vi "Pack for gRPC.vi"(8 "error in":errorcluster, 9 "configuration / results":enum16{"Configuration", "Results"}(ring), 10 "data value":variant, 11 "measurement plugin service in":refnum<class "Measurement Plugin Service.lvclass">) -> (0 "error out":errorcluster, 2 "any":T1, 3 "measurement plugin service out":refnum<class "Measurement Plugin Service.lvclass">)   [LabVIEW 2021, in "NI Measurement Plug-In SDK.lvlib" / "Measurement Plugin Service.lvclass"]
uses:
  Measurement Plugin Service.lvclass
  <vilib>/gRPC/LabVIEW gRPC Library/Shared/Any.ctl
  <vilib>/gRPC/LabVIEW gRPC Library/grpc-lvsupport-release.lvlib
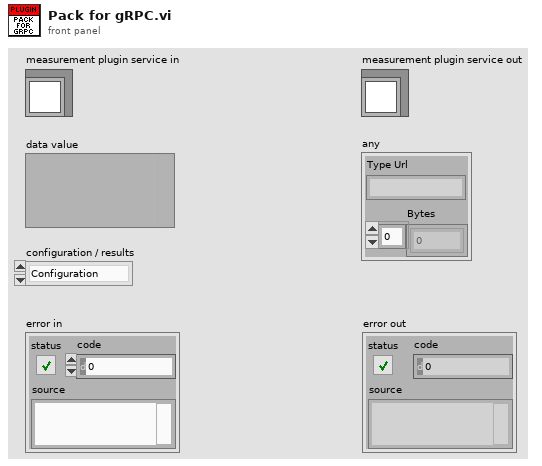
[diagram p1: front panel]
types:
  T1 = typedef "grpc-lvsupport-release.lvlib/Any.ctl" = cluster{"Type Url":string, "Bytes":u8[]}
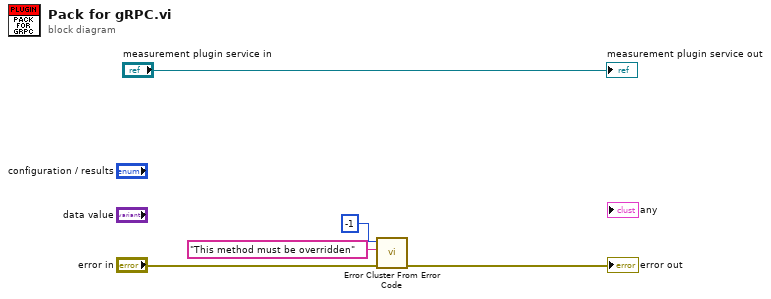
[diagram p0: block diagram]
diagram:
  n1 = call <vilib>:"Error Cluster From Error Code.vi"("error in (no error)"="error in", "error message (\"\")"="This method must be overridden" ("error message (\"\")"), "error code (0)"=-1) -> ("error out"=→"error out":errorcluster)  [unwired: 6 in]
  "measurement plugin service out" <- "measurement plugin service in"
